vi "Configure Alarm.vi"(0 "VISA resource name":refnum<visa-resource-name>, 1 "High Value (0.00000)":dbl format="%.5f", 2 "Low Value (0.00000)":dbl format="%.5f", 5 "Input (0:A)":u16(ring) items=["A", "B", "C", "D"], 7 "Enable Alarm (F: Off)":bool, 9 "Enable Latching (F: Off)":bool, 11 "error in (no error)":errorcluster, 12 "Enable Beep (F: Off)":bool, 13 "Enable Display (F: Off)":bool, 14 "Deadband (0.00000)":dbl format="%.5f") -> (4 "VISA resource name out":refnum<visa-resource-name>, 15 "error out":errorcluster)   [LabVIEW 2013, in "Lake Shore 336.lvlib"]
doc: "This VI configures the input alarm settings. Each input of the Model 336 has high and low alarm capability. Input reading data from any source can be compared to the alarm setpoint values. A reading higher than the high alarm setpoint triggers the high alarm for that input. A reading lower than the low alarm setpoint triggers the low alarm for that input."
uses:
  Lake Shore 336.lvlib
  Instance           1 23Saved   Configure Alarm .vi
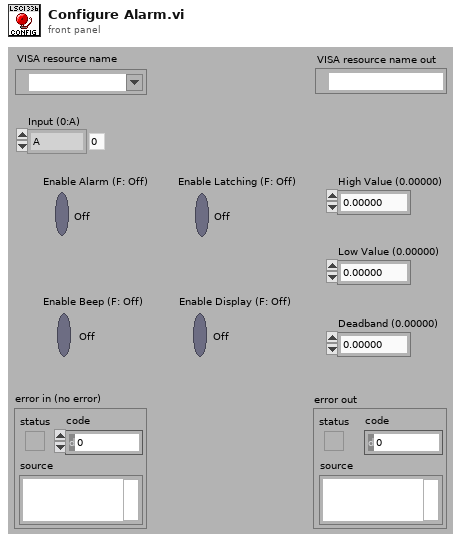
[diagram p1: front panel]
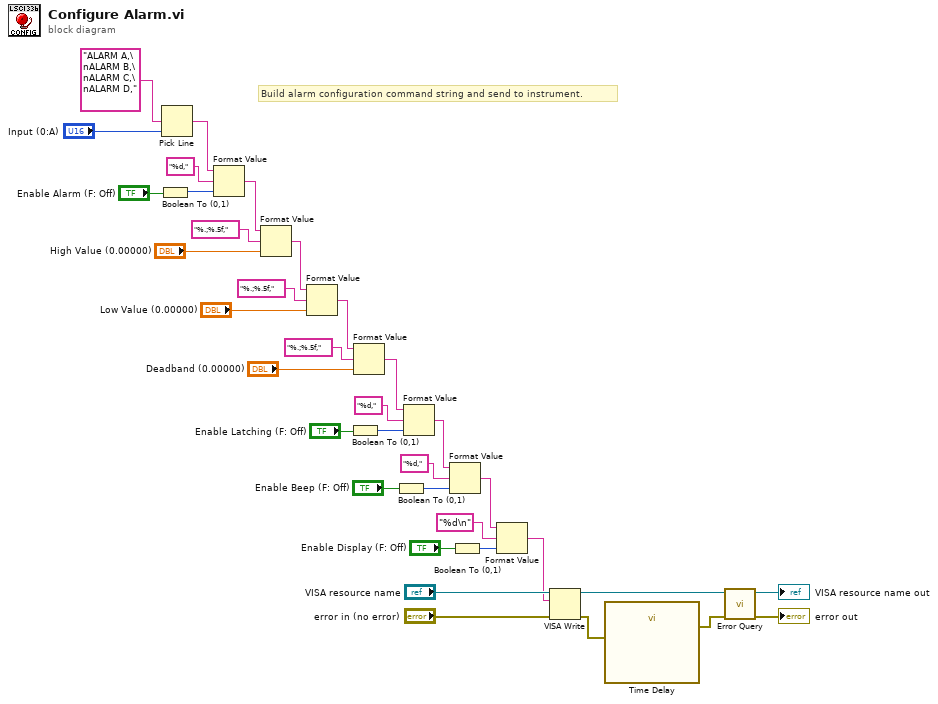
[diagram p0: block diagram]
diagram:
  # "Build alarm configuration command string and send to instrument."
  n1 = Boolean To (0,1)(Boolean="Enable Alarm (F: Off)") -> (0, 1=w27:i16)
  n2 = Pick Line(multi-line string="ALARM A,\nALARM B,\nALARM C,\nALARM D,", line index="Input (0:A)") -> (output string=w11:string)  [unwired: 1 in]
  n3 = Format Value(string ("")=w11, format string="%d,", value (0)=w27) -> (output string=w10:string)
  n4 = Format Value(string ("")=w10, format string="%.;%.5f,", value (0)="High Value (0.00000)") -> (output string=w9:string)
  n5 = Format Value(string ("")=w9, format string="%.;%.5f,", value (0)="Low Value (0.00000)") -> (output string=w8:string)
  n6 = Boolean To (0,1)(Boolean="Enable Latching (F: Off)") -> (0, 1=w23:i16)
  n7 = Format Value(string ("")=w8, format string="%.;%.5f,", value (0)="Deadband (0.00000)") -> (output string=w7:string)
  n8 = Boolean To (0,1)(Boolean="Enable Beep (F: Off)") -> (0, 1=w4:i16)
  n9 = Format Value(string ("")=w7, format string="%d,", value (0)=w23) -> (output string=w3:string)
  n10 = Format Value(string ("")=w3, format string="%d,", value (0)=w4) -> (output string=w1:string)
  n11 = Boolean To (0,1)(Boolean="Enable Display (F: Off)") -> (0, 1=w13:i16)
  n12 = Format Value(string ("")=w1, format string="%d\n", value (0)=w13) -> (output string=w6:string)
  n13 = VISA Write(VISA resource name="VISA resource name", write buffer=w6, error in (no error)="error in (no error)") -> (VISA resource name out=w33:refnum<visa-resource-name>, error out=w21:errorcluster)  [unwired: 1 out]
  n14 = call "Time Delay"("error in (no error)"=w21) -> ("error out"=w20:errorcluster)  [unwired: 10 in]
  n15 = call "Error Query.vi"("error in (no error)"=w20, "VISA resource name"=w33) -> ("error out"=→"error out":errorcluster, "VISA resource name out"=→"VISA resource name out":refnum<visa-resource-name>)  [unwired: 7 in, 1 out]
